vi "AFG3352XGUI.panel.vi"() -> ()   [LabVIEW 2014, in "AFG3352XGUI.lvlib"]
doc: "GUI for the AFGBase class (and its children)\n\nauthor: Dietrich Beck, GSI\nlicense: GPL"
uses:
  AFG3352XGUI.lvlib
  CSlibraries-extern/DimLVEvent/DimIndicators/DimIndicators.numericType.ctl
  CSlibraries-extern/DimLVEvent/DimIndicators/DimIndicators.anyType.ctl
  CSlibraries/UtilityLib/UtilityLib.valueStatus.ctl
  CSlibraries/UtilityLib/UtilityLib.helpType.ctl
  CSCore/CSSystem/CoreLib/CoreLib.int 2 byte array.vi
  CSCore/CSSystem/CoreLib/CoreLib.short 2 byte array.vi
  CSCore/CSSystem/CoreLib/CoreLib.short array 2 byte array.vi
  CSCore/CSSystem/CoreLib/CoreLib.double 2 byte array.vi
  CSCore/CSSystem/CoreLib/CoreLib.lvlib
  CSCore/CSObj/CSObj.lvlib
  CSlibraries/UtilityLib/UtilityLib.lvlib
  CSCore/CSApplicationBaseClasses/DeviceBase/DeviceBase.lvlib
  CSlibraries-extern/DimLVEvent/DimIndicators/DimIndicators.lvlib
  CSCore/GUIs/GOGUserGUIs/DeviceBaseGUI/DeviceBaseGUI.lvlib
panel:
  in  "actBurstMode 2":T1 caption="dic_service_numeric"
  in  "actBurstMode":T1 caption="dic_service_numeric"
  in  "actMode2":T1 caption="dic_service_numeric"
  in  "actMode":T1 caption="dic_service_numeric"
  in  "actOffset2":T1 caption="dic_service_numeric"
  in  "actAmplitude2":T1 caption="dic_service_numeric"
  in  "actPhase2":T1 caption="dic_service_numeric"
  in  "actFrequency2":T1 caption="dic_service_numeric"
  in  "Set":bool
  in  "inc":dbl
  in  "setValue":dbl
  out "Busy":bool
  out "ErrorString":string
  in  "nomValue":T1 caption="dic_service_numeric"
  in  "actOffset":T1 caption="dic_service_numeric"
  in  "actAmplitude":T1 caption="dic_service_numeric"
  in  "actPhase":T1 caption="dic_service_numeric"
  in  "actFrequency":T1 caption="dic_service_numeric"
  out "deviceIDString":string
  in  "tab":enum32{"standard", "advanced"}(tab)
  out "channelIndex":u16
  in  "nextChannel":bool
  in  "previousChannel":bool
  in  "listbox":i32(listbox)
  in  "function":u16(ring) items=["choose function", "SetFrequency", "SetAmplitude", "SetPhase", "SetDCOffset", "SetOutputEnabled", "SetMode", "SetTrigger", "SetBurstMode", "Reset"]
  in  "advancedGUI":bool
  in  "minus":bool
  in  "plus":bool
  out "loop counter":i32
  out "error out":errorcluster
  in  "error in (no error)":errorcluster
  in  "object ref":refnum<vi>
  in  "state":T1 caption="dic_service_numeric"
  in  "deviceID":T2 caption="dic_service_anyType"
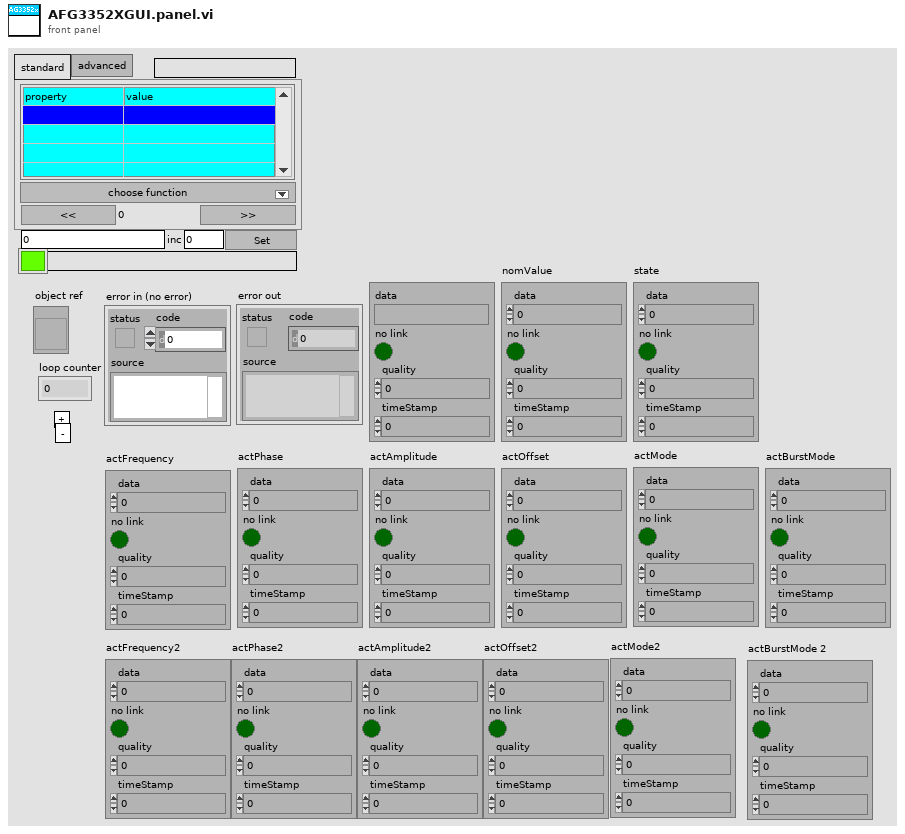
[diagram p1: front panel]
types:
  T1 = typedef "DimIndicators.lvlib/DimIndicators.numericType.ctl" = cluster{"data":dbl, "no link":bool, "quality":i32, "timeStamp":dbl}
  T2 = typedef "DimIndicators.lvlib/DimIndicators.anyType.ctl" = cluster{"data":string, "no link":bool, "quality":i32, "timeStamp":dbl}
  T3 = typedef "UtilityLib.lvlib/UtilityLib.valueStatus.ctl" = enum16{"no info available", "stand by/off", "on", "warning", "alarm/malfunction", "not implemented", "user action required", "important information", "system default", "control default", "indicator default", "button default"}
  T4 = typedef "UtilityLib.lvlib/UtilityLib.helpType.ctl" = enum16{"unknown", "menu", "description", "about", "special0", "special1", "special2"}
  T5 = typedef "CoreDefs.rawDataType.ctl" = i8[]
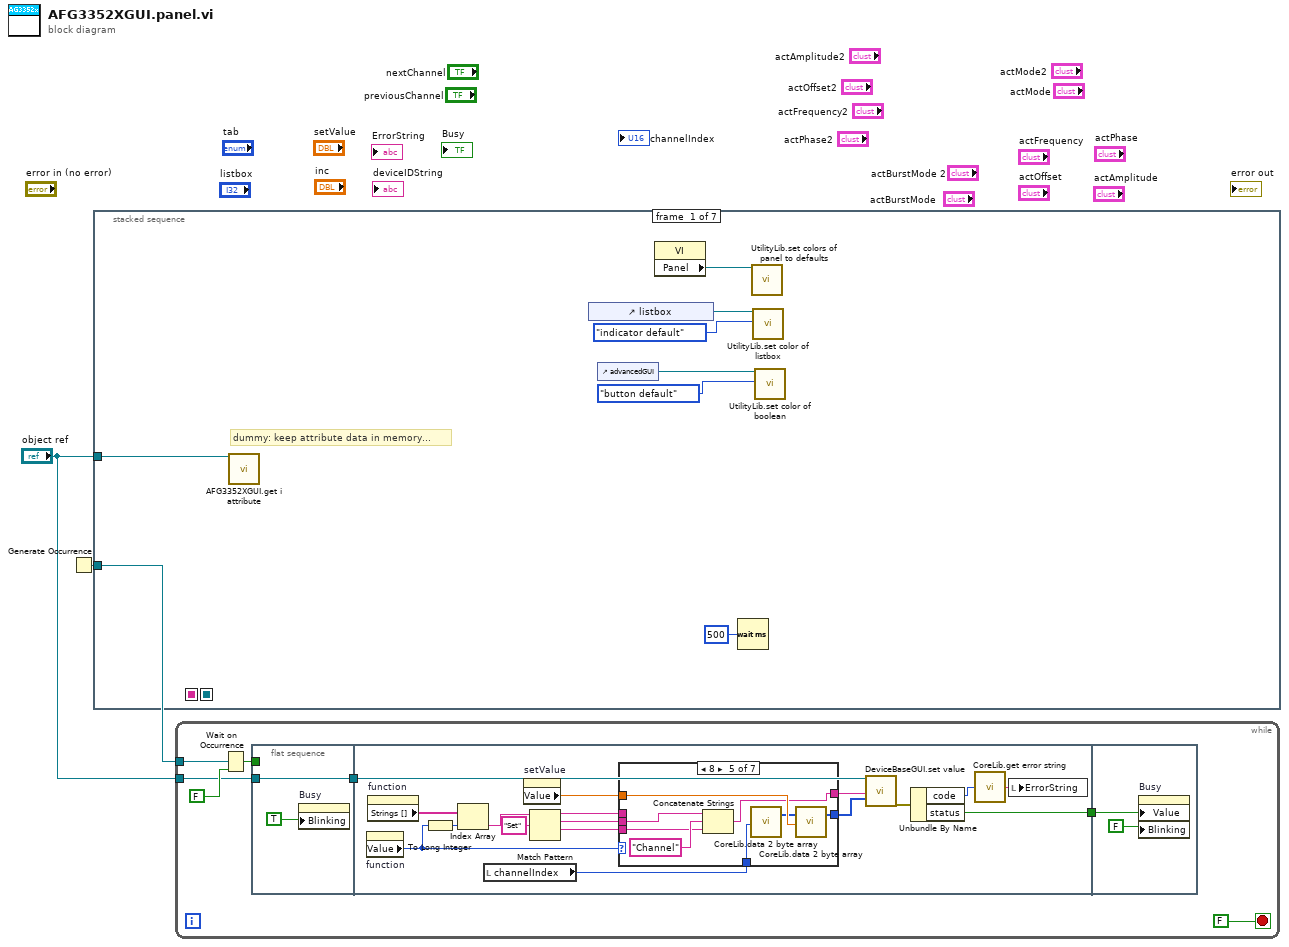
[diagram p0: block diagram]
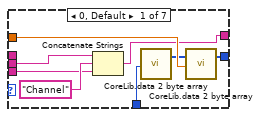
[diagram p2: hidden frame]
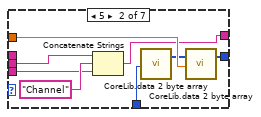
[diagram p3: hidden frame]
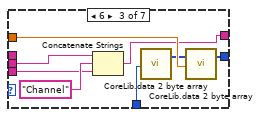
[diagram p4: hidden frame]
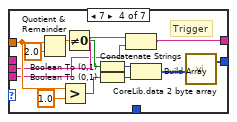
[diagram p5: hidden frame]
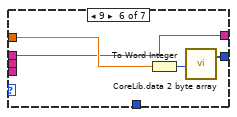
[diagram p6: hidden frame]
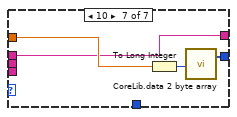
[diagram p7: hidden frame]
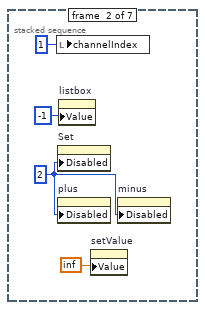
[diagram p8: hidden frame]
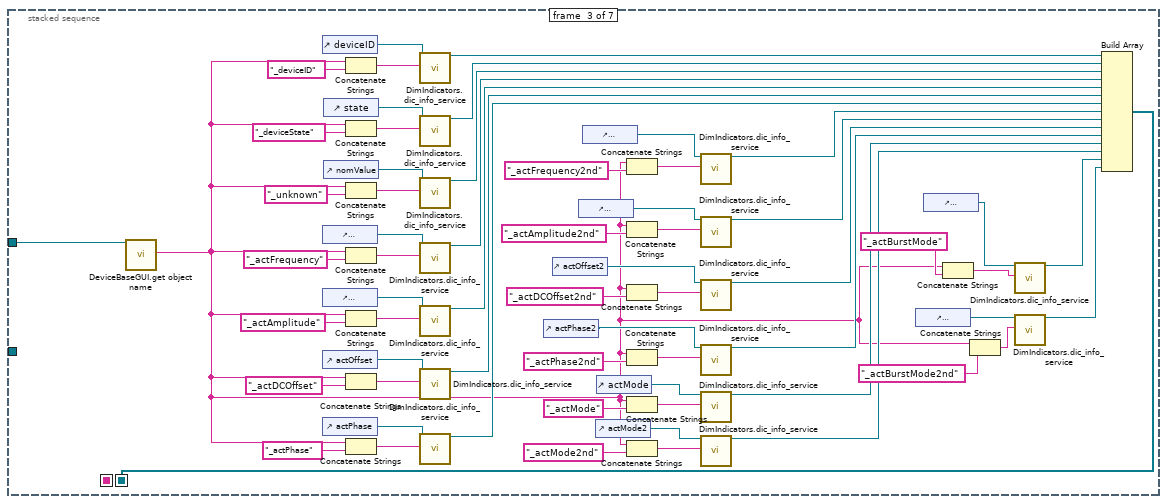
[diagram p9: hidden frame]
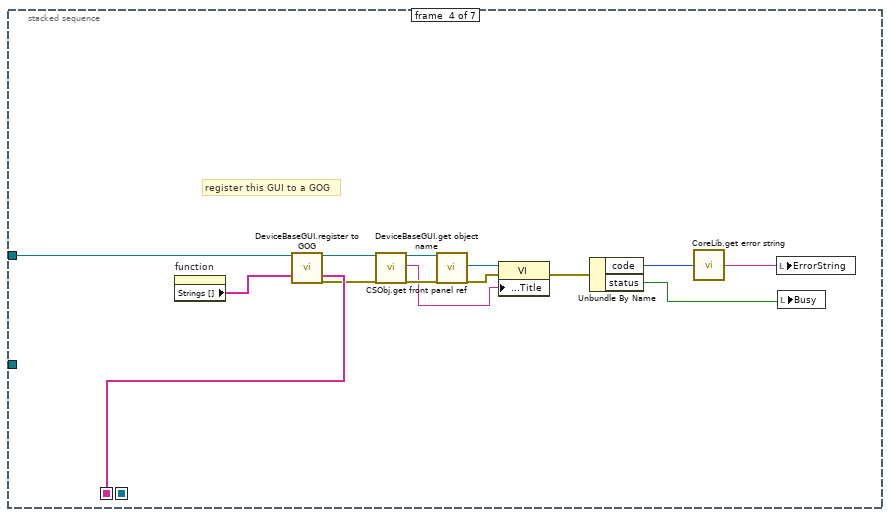
[diagram p10: hidden frame]
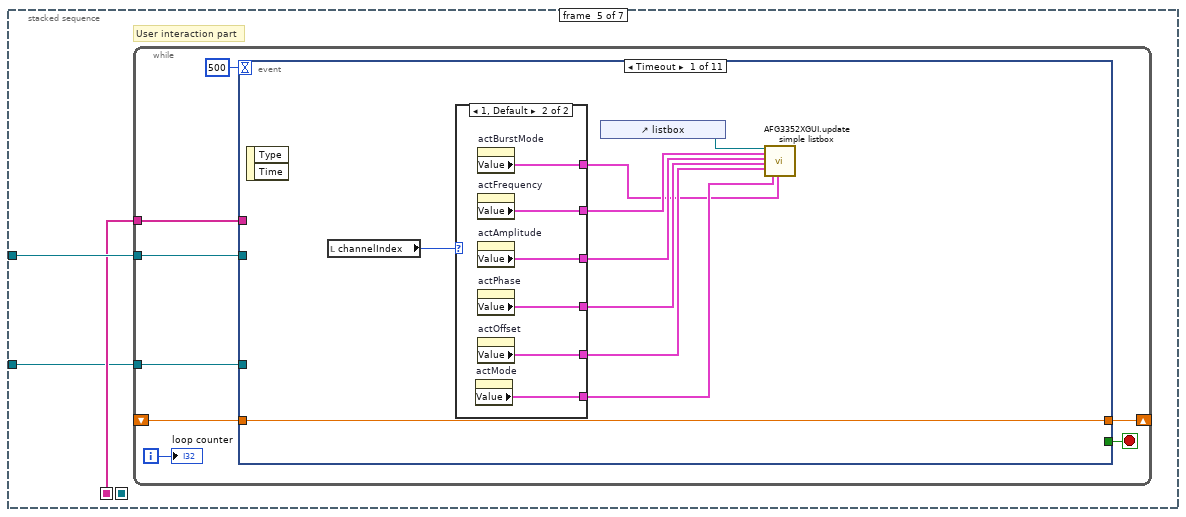
[diagram p11: hidden frame]
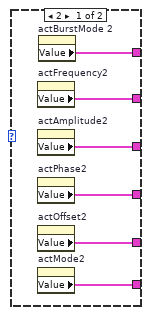
[diagram p12: hidden frame]
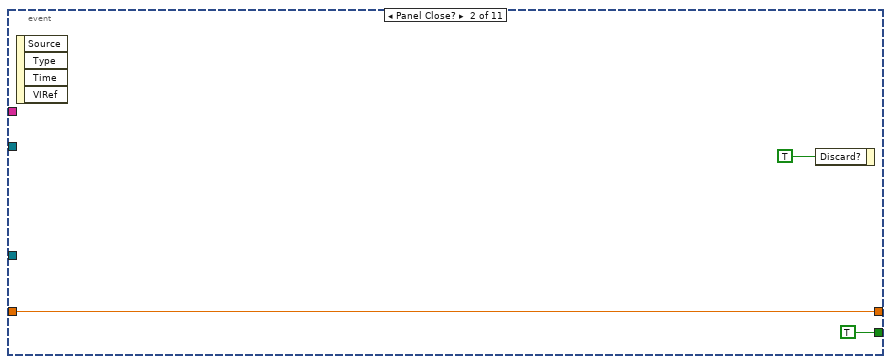
[diagram p13: hidden frame]
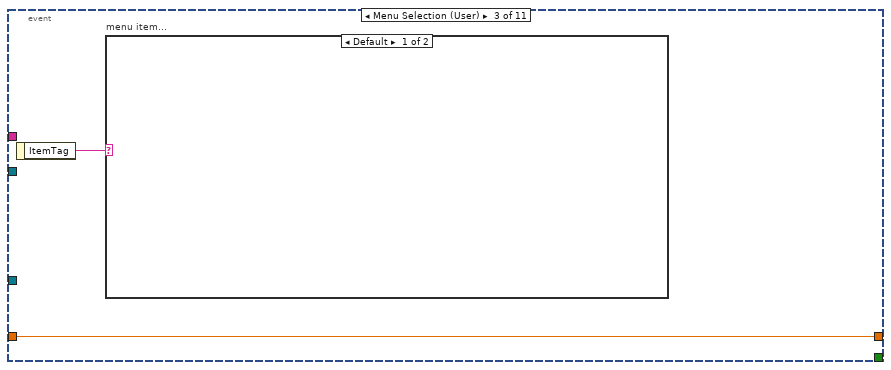
[diagram p14: hidden frame]
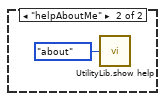
[diagram p15: hidden frame]
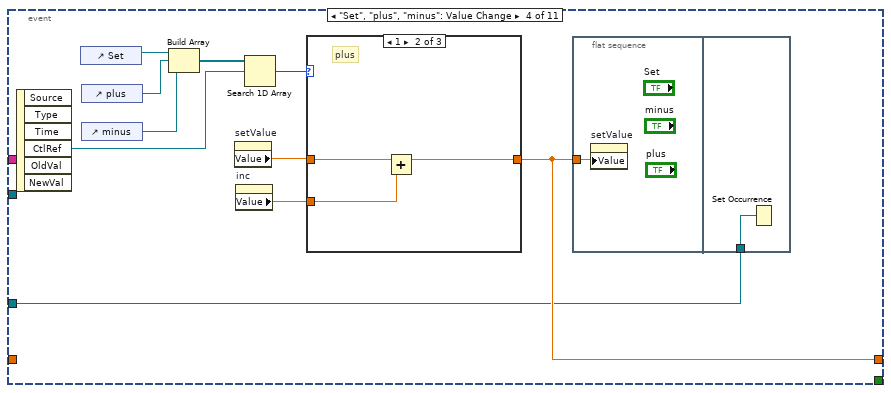
[diagram p16: hidden frame]
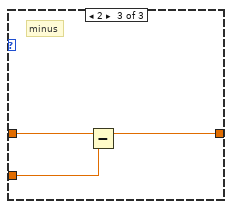
[diagram p18: hidden frame]
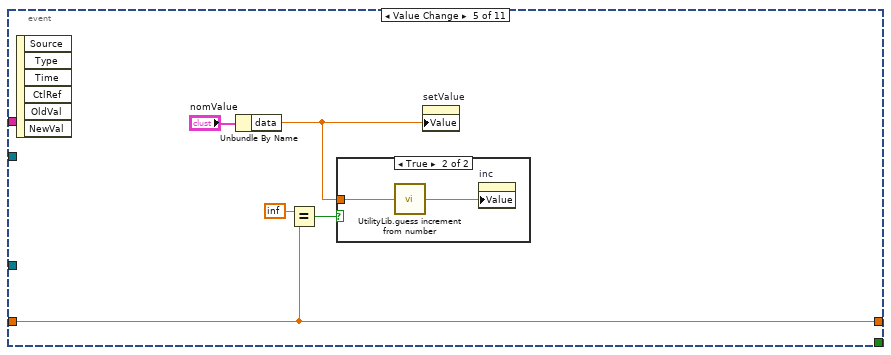
[diagram p19: hidden frame]
diagram:
  n1 = Generate Occurrence() -> (w1:refnum<k4>)
  n2 = stacked-sequence {
    seq-local: [_ _ _ w88 _ _ _] -> [_ _ _ _ w92 _ _]
    seq-local: [_ _ w47 _ _ _ _] -> [_ _ _ _ _ w216 _]
    tunnel: "object ref" -> [w3 _ w76 w78 w93 _ w218]
    tunnel: w1 -> [_ _ _ _ w91 _ _]
    frame #0 {
      # "dummy: keep attribute data in memory..."
      n3 = call "AFG3352XGUI.get i attribute.vi"("i ref in"=w3) -> ()  [unwired: 16 in, 3 out]
      n4 = control-ref of="listbox"() -> (w7:refnum<vi>)
      n5 = control-ref of="advancedGUI"() -> (w5:refnum<vi>)
      n6 = property class="VI"() -> ("Panel"=w8:refnum<vi>)  [unwired: 2 in, 2 out]
      n7 = Wait (ms)(milliseconds to wait=u32 500) -> ()  [unwired: 1 out]
      n8 = call "UtilityLib.set colors of panel to defaults.vi"("Front Panel"=w8) -> ()  [unwired: 18 in, 1 out]
      n9 = call "UtilityLib.set color of listbox.vi"("listboxRef"=w7, "valueStatus"=UtilityLib.valueStatus."indicator default") -> ()  [unwired: 17 in, 1 out]
      n10 = call "UtilityLib.set color of boolean.vi"("button"=w5, "valueStatus"=UtilityLib.valueStatus."button default") -> ()  [unwired: 17 in, 1 out]
    }
    frame #1 {
      w13 = u8 2 ("Disabled")
      n11 = local write "channelIndex"(u16 1 ("channelIndex")) -> ()
      n12 = property on="Set" class="Bool"("Disabled"=w13) -> ()  [unwired: 2 in, 2 out]
      n13 = property on="plus" class="Bool"("Disabled"=w13) -> ()  [unwired: 2 in, 2 out]
      n14 = property on="listbox" class="MCListbox (strict)"("Value"=-1 ("listbox")) -> ()  [unwired: 2 in, 2 out]
      n15 = property on="setValue" class="DigNum (strict)"("Value"=inf) -> ()  [unwired: 2 in, 2 out]
      n16 = property on="minus" class="Bool"("Disabled"=w13) -> ()  [unwired: 2 in, 2 out]
    }
    frame #2 {
      n17 = call "DeviceBaseGUI.get object name.vi"("i ref in"=w76) -> ("objectName"=w14:string)  [unwired: 16 in, 2 out]
      n18 = control-ref of="deviceID"() -> (w67:refnum<vi>)
      n19 = control-ref of="actFrequency"() -> (w58:refnum<vi>)
      n20 = control-ref of="actAmplitude"() -> (w57:refnum<vi>)
      n21 = control-ref of="actOffset"() -> (w56:refnum<vi>)
      n22 = control-ref of="actPhase"() -> (w55:refnum<vi>)
      n23 = control-ref of="state"() -> (w60:refnum<vi>)
      n24 = control-ref of="nomValue"() -> (w59:refnum<vi>)
      n25 = Concatenate Strings(w14, "_deviceID" ("string")) -> (w68:string)
      n26 = Concatenate Strings(w14, "_deviceState" ("string")) -> (w61:string)
      n27 = Concatenate Strings(w14, "_unknown" ("string")) -> (w62:string)
      n28 = Concatenate Strings(w14, "_actFrequency" ("string")) -> (w63:string)
      n29 = Concatenate Strings(w14, "_actAmplitude" ("string")) -> (w64:string)
      n30 = Concatenate Strings(w14, "_actDCOffset" ("string")) -> (w65:string)
      n31 = Concatenate Strings(w14, "_actPhase" ("string")) -> (w66:string)
      n32 = call "DimIndicators.dic_info_service.vi"("controlRef"=w67, "serviceName"=w68) -> ("controlRef out"=w54:refnum<vi>)  [unwired: 16 in, 1 out]
      n33 = call "DimIndicators.dic_info_service.vi"("controlRef"=w60, "serviceName"=w61) -> ("controlRef out"=w53:refnum<vi>)  [unwired: 16 in, 1 out]
      n34 = call "DimIndicators.dic_info_service.vi"("controlRef"=w59, "serviceName"=w62) -> ("controlRef out"=w52:refnum<vi>)  [unwired: 16 in, 1 out]
      n35 = call "DimIndicators.dic_info_service.vi"("controlRef"=w58, "serviceName"=w63) -> ("controlRef out"=w51:refnum<vi>)  [unwired: 16 in, 1 out]
      n36 = call "DimIndicators.dic_info_service.vi"("controlRef"=w57, "serviceName"=w64) -> ("controlRef out"=w50:refnum<vi>)  [unwired: 16 in, 1 out]
      n37 = call "DimIndicators.dic_info_service.vi"("controlRef"=w56, "serviceName"=w65) -> ("controlRef out"=w49:refnum<vi>)  [unwired: 16 in, 1 out]
      n38 = call "DimIndicators.dic_info_service.vi"("controlRef"=w55, "serviceName"=w66) -> ("controlRef out"=w48:refnum<vi>)  [unwired: 16 in, 1 out]
      n39 = control-ref of="actPhase2"() -> (w24:refnum<vi>)
      n40 = control-ref of="actOffset2"() -> (w23:refnum<vi>)
      n41 = control-ref of="actAmplitude2"() -> (w33:refnum<vi>)
      n42 = control-ref of="actFrequency2"() -> (w34:refnum<vi>)
      n43 = control-ref of="actMode2"() -> (w25:refnum<vi>)
      n44 = control-ref of="actMode"() -> (w26:refnum<vi>)
      n45 = Concatenate Strings(w14, "_actFrequency2nd" ("string")) -> (w42:string)
      n46 = Concatenate Strings(w14, "_actAmplitude2nd" ("string")) -> (w41:string)
      n47 = Concatenate Strings(w14, "_actDCOffset2nd" ("string")) -> (w40:string)
      n48 = Concatenate Strings(w14, "_actPhase2nd" ("string")) -> (w39:string)
      n49 = Concatenate Strings(w14, "_actMode" ("string")) -> (w31:string)
      n50 = Concatenate Strings(w14, "_actMode2nd" ("string")) -> (w29:string)
      n51 = call "DimIndicators.dic_info_service.vi"("controlRef"=w34, "serviceName"=w42) -> ("controlRef out"=w35:refnum<vi>)  [unwired: 16 in, 1 out]
      n52 = call "DimIndicators.dic_info_service.vi"("controlRef"=w33, "serviceName"=w41) -> ("controlRef out"=w36:refnum<vi>)  [unwired: 16 in, 1 out]
      n53 = call "DimIndicators.dic_info_service.vi"("controlRef"=w23, "serviceName"=w40) -> ("controlRef out"=w37:refnum<vi>)  [unwired: 16 in, 1 out]
      n54 = call "DimIndicators.dic_info_service.vi"("controlRef"=w24, "serviceName"=w39) -> ("controlRef out"=w38:refnum<vi>)  [unwired: 16 in, 1 out]
      n55 = call "DimIndicators.dic_info_service.vi"("controlRef"=w26, "serviceName"=w31) -> ("controlRef out"=w28:refnum<vi>)  [unwired: 16 in, 1 out]
      n56 = call "DimIndicators.dic_info_service.vi"("controlRef"=w25, "serviceName"=w29) -> ("controlRef out"=w27:refnum<vi>)  [unwired: 16 in, 1 out]
      n57 = control-ref of="actBurstMode 2"() -> (w19:refnum<vi>)
      n58 = control-ref of="actBurstMode"() -> (w20:refnum<vi>)
      n59 = Concatenate Strings(w14, "_actBurstMode" ("string")) -> (w16:string)
      n60 = Concatenate Strings(w14, "_actBurstMode2nd" ("string")) -> (w18:string)
      n61 = call "DimIndicators.dic_info_service.vi"("controlRef"=w20, "serviceName"=w16) -> ("controlRef out"=w22:refnum<vi>)  [unwired: 16 in, 1 out]
      n62 = call "DimIndicators.dic_info_service.vi"("controlRef"=w19, "serviceName"=w18) -> ("controlRef out"=w21:refnum<vi>)  [unwired: 16 in, 1 out]
      n63 = Build Array(w54, w53, w52, w51, w50, w49, w48, w35, w36, w37, w38, w28, w27, w22, w21) -> (w47:refnum<vi>[])
    }
    frame #3 {
      # "register this GUI to a GOG"
      n64 = property on="function" class="Ring (strict)"() -> ("Strings []"=w89:string[])  [unwired: 2 in, 2 out]
      n65 = call "DeviceBaseGUI.register to GOG.vi"("i ref in"=w78, "myMethods"=w89) -> ("i ref out"=w86:refnum<vi>, "configuredMethods"=w88:string[], "error out"=w87:errorcluster)  [unwired: 15 in]
      n66 = call "DeviceBaseGUI.get object name.vi"("i ref in"=w86, "error in (no error)"=w87) -> ("i ref out"=w85:refnum<vi>, "objectName"=w77:string, "error out"=w84:errorcluster)  [unwired: 15 in]
      n67 = call "CSObj.get front panel ref.vi"("i ref in"=w85, "error in (no error)"=w84) -> ("frontPanelRef"=w90:refnum<vi>, "error out"=w80:errorcluster)  [unwired: 15 in, 1 out]
      n68 = property class="VI"(reference=w90, error in=w80, "Front Panel Window:Title"=w77) -> (error out=w79:errorcluster)  [unwired: 1 out]
      n69 = Unbundle By Name(w79) -> ("code"=w83:i32, "status"=w81:bool)
      n70 = call "CoreLib.get error string.vi"("Error Code"=w83) -> ("Error String"=w82:string)
      n71 = local write "ErrorString"(w82) -> ()
      n72 = local write "Busy"(w81) -> ()
    }
    frame #4 {
      # "User interaction part"
      n73 = while {
        tunnel: w93 -> [w100]
        shift-right: [w97] -> _
        shift-left: _ -> [w98]
        tunnel: w92 -> [w96]
        tunnel: w91 -> [w95]
        i -> [w101]
        stop <- w94 stop-if-true
        n74 = event shown="[0] Timeout" {
          selector: _ -> [_ _ _ _ _ _ _ _ _ _ _]
          dyn-events: _ -> [_ _ _ _ _ _ _ _ _ _ _]
          timeout: 500 -> [_ _ _ _ _ _ _ _ _ _ _]
          tunnel: w100 -> [_ _ _ _ _ w165 _ _ w195 _ _]
          tunnel: [w110 w125 w127 w130 w150 w156 w185 w191 w194 w205 w214] -> w97
          tunnel: w98 -> [w110 w125 w127 _ w150 _ w185 w191 w194 w205 w214]
          tunnel: w96 -> [_ _ _ _ _ w163 _ _ _ _ _]
          tunnel: w95 -> [_ _ _ w129 _ _ _ _ _ _ _]
          tunnel: [_ TRUE ("Discard?") _ _ _ _ _ _ _ _ _] -> w94
          event Timeout {
            n75 = event-data() -> ()  [unwired: 1 in, 2 out]
            n76 = local read "channelIndex"() -> (w104:u16)
            n77 = case shown="1, Default" w104 {
              tunnel: [w116 w122] -> w108
              tunnel: [w115 w121] -> w107
              tunnel: [w114 w120] -> w106
              tunnel: [w113 w119] -> w105
              tunnel: [w112 w118] -> w103
              tunnel: [w111 w117] -> w102
              frame 2 {
                n78 = property on="actFrequency2" class="Clust (strict)"() -> ("Value"=w116:T1)  [unwired: 2 in, 2 out]
                n79 = property on="actAmplitude2" class="Clust (strict)"() -> ("Value"=w115:T1)  [unwired: 2 in, 2 out]
                n80 = property on="actPhase2" class="Clust (strict)"() -> ("Value"=w114:T1)  [unwired: 2 in, 2 out]
                n81 = property on="actOffset2" class="Clust (strict)"() -> ("Value"=w113:T1)  [unwired: 2 in, 2 out]
                n82 = property on="actMode2" class="Clust (strict)"() -> ("Value"=w112:T1)  [unwired: 2 in, 2 out]
                n83 = property on="actBurstMode 2" class="Clust (strict)"() -> ("Value"=w111:T1)  [unwired: 2 in, 2 out]
              }
              frame 1, Default {
                n84 = property on="actMode" class="Clust (strict)"() -> ("Value"=w118:T1)  [unwired: 2 in, 2 out]
                n85 = property on="actBurstMode" class="Clust (strict)"() -> ("Value"=w117:T1)  [unwired: 2 in, 2 out]
                n86 = property on="actFrequency" class="Clust (strict)"() -> ("Value"=w122:T1)  [unwired: 2 in, 2 out]
                n87 = property on="actAmplitude" class="Clust (strict)"() -> ("Value"=w121:T1)  [unwired: 2 in, 2 out]
                n88 = property on="actPhase" class="Clust (strict)"() -> ("Value"=w120:T1)  [unwired: 2 in, 2 out]
                n89 = property on="actOffset" class="Clust (strict)"() -> ("Value"=w119:T1)  [unwired: 2 in, 2 out]
              }
            }
            n90 = control-ref of="listbox"() -> (w109:refnum<vi>)
            n91 = call "AFG3352XGUI.update simple listbox.vi"("listbox"=w109, "actFrequency"=w108, "actAmplitude"=w107, "actPhase"=w106, "actOffset"=w105, "actMode"=w103, "actBurstMode"=w102) -> ()  [unwired: 12 in, 1 out]
          }
          event Panel Close? {
            n92 = event-data() -> ()  [unwired: 1 in, 4 out]
            n93 = event-data("Discard?"=TRUE) -> ()  [unwired: 1 in, 1 out]
          }
          event Menu Selection (User) {
            n94 = event-data() -> ("ItemTag"=w126:string)  [unwired: 1 in]
            n95 = case "menu item..." shown="Default" w126 {
              frame Default {
              }
              frame "helpAboutMe" {
                n96 = call "UtilityLib.show help.vi"("helpType"=UtilityLib.helpType."about") -> ()
              }
            }
          }
          event "Set", "plus", "minus": Value Change {
            n97 = event-data() -> ("CtlRef"=w134:refnum<vi>)  [unwired: 1 in, 5 out]
            n98 = control-ref of="Set"() -> (w138:refnum<vi>)
            n99 = control-ref of="plus"() -> (w137:refnum<vi>)
            n100 = control-ref of="minus"() -> (w136:refnum<vi>)
            n101 = Build Array(w138, w137, w136) -> (w135:refnum<vi>[])
            n102 = property on="setValue" class="DigNum (strict)"() -> ("Value"=w131:dbl)  [unwired: 2 in, 2 out]
            n103 = property on="inc" class="DigNum (strict)"() -> ("Value"=w132:dbl)  [unwired: 2 in, 2 out]
            n104 = Search 1D Array(1D array=w135, element=w134) -> (index of element=w133:i32)  [unwired: 1 in]
            n105 = case shown="1" w133 {
              tunnel: [w141 w143 w146] -> w130
              tunnel: w131 -> [w141 w144 w147]
              tunnel: w132 -> [_ w142 w145]
              frame 0, Default {
                # "set"
              }
              frame 1 {
                # "plus"
                n106 = Add(x=w144, y=w142) -> (x+y=w143:dbl)
              }
              frame 2 {
                # "minus"
                n107 = Subtract(x=w147, y=w145) -> (x-y=w146:dbl)
              }
            }
            n108 = flat-sequence {
              tunnel: w130 -> [w139]
              tunnel: w129 -> [w140]
              frame #0 {
                n109 = property on="setValue" class="DigNum (strict)"("Value"=w139) -> ()  [unwired: 2 in, 2 out]
              }
              frame #1 {
                n110 = Set Occurrence(w140) -> ()
              }
            }
          }
          event Value Change {
            n111 = event-data() -> ()  [unwired: 1 in, 6 out]
            n112 = Unbundle By Name("nomValue") -> ("data"=w152:dbl)
            n113 = Equal?(x=inf, y=w150) -> (x = y?=w148:bool)
            n114 = case shown="True" w148 {
              tunnel: w152 -> [_ w154]
              frame False {
              }
              frame True {
                n115 = call "UtilityLib.guess increment from number.vi"("number"=w154) -> ("increment"=w153:dbl)
                n116 = property on="inc" class="DigNum (strict)"("Value"=w153) -> ()  [unwired: 2 in, 2 out]
              }
            }
            n117 = property on="setValue" class="DigNum (strict)"("Value"=w152) -> ()  [unwired: 2 in, 2 out]
          }
          event "function": Value Change {
            w156 = inf
            n118 = event-data() -> ()  [unwired: 1 in, 6 out]
            n119 = property on="function" class="Ring (strict)"() -> ("Strings []"=w164:string[])  [unwired: 2 in, 2 out]
            n120 = property on="setValue" class="DigNum (strict)"("Value"=w156) -> (error out=w160:errorcluster)  [unwired: 2 in, 1 out]
            n121 = control-ref of="nomValue"() -> (w157:refnum<vi>)
            n122 = To Long Integer(number="function") -> (32bit integer=w155:i32)
            n123 = Index Array(array=w164, index=w155) -> (element=w162:string)
            n124 = call "DimIndicators.dic_release_service.vi"("controlRef"=w157) -> ("error out"=w158:errorcluster)  [unwired: 18 in]
            n125 = Search 1D Array(1D array=w163, element=w162) -> (index of element=w161:i32)  [unwired: 1 in]
            n126 = case "method configured?" shown="0, Default" w161 {
              tunnel: w165 -> [w172 _]
              tunnel: "function" -> [w171 _]
              tunnel: w158 -> [w169 _]
              tunnel: w160 -> [_ _]
              tunnel: w157 -> [w168 _]
              frame 0, Default {
                w170 = u8 0 ("Disabled")
                n127 = case shown="6" w171 {
                  tunnel: ["_nomFrequency" "_nomAmplitude" "_nomPhase" "_nomDCOffset" "_nomOutputEnabled" "_nomWaveformType" "unknown"] -> w173
                  frame 1 {
                  }
                  frame 2 {
                  }
                  frame 3 {
                  }
                  frame 4 {
                  }
                  frame 6 {
                  }
                  frame 7 {
                  }
                  frame 0, Default {
                  }
                }
                n128 = call "DeviceBaseGUI.get object name.vi"("i ref in"=w172) -> ("objectName"=w166:string)  [unwired: 16 in, 2 out]
                n129 = Concatenate Strings(w166, w173) -> (w167:string)
                n130 = property on="Set" class="Bool"("Disabled"=w170) -> ()  [unwired: 2 in, 2 out]
                n131 = property on="plus" class="Bool"("Disabled"=w170) -> ()  [unwired: 2 in, 2 out]
                n132 = call "DimIndicators.dic_info_service.vi"("controlRef"=w168, "serviceName"=w167, "error in (no error)"=w169) -> ()  [unwired: 15 in, 2 out]
                n133 = property on="minus" class="Bool"("Disabled"=w170) -> ()  [unwired: 2 in, 2 out]
              }
              frame -1 {
                w181 = u8 2 ("Disabled")
                n134 = property on="Set" class="Bool"("Disabled"=w181) -> ()  [unwired: 2 in, 2 out]
                n135 = property on="plus" class="Bool"("Disabled"=w181) -> ()  [unwired: 2 in, 2 out]
                n136 = property on="minus" class="Bool"("Disabled"=w181) -> ()  [unwired: 2 in, 2 out]
              }
            }
          }
          event Value Change {
            n137 = event-data() -> ()  [unwired: 1 in, 6 out]
            n138 = Unbundle By Name("deviceID") -> ("data"=w184:string)
            n139 = call "UtilityLib.remove white spaces.vi"("string with blanks"=w184) -> ("string without white spaces"=w183:string)  [unwired: 14 in, 4 out]
            n140 = property on="deviceIDString" class="Str"("Value"=w183) -> ()  [unwired: 2 in, 2 out]
          }
          event Value Change {
            n141 = event-data() -> ()  [unwired: 1 in, 6 out]
            n142 = Unbundle By Name("state") -> ("no link"=w192:bool, "data"=w188:dbl)
            n143 = call "DeviceBase.device state 2 value status.vi"("deviceState"=w188, "no link"=w192) -> ("valueStatus"=w190:T3)
            n144 = call "UtilityLib.Sixcolor.vi"("State"=w190) -> ("elementBackground"=w189:u32, "elementText"=w186:u32)  [unwired: 2 in, 2 out]
            n145 = property on="deviceIDString" class="Str"("Text.BGColor"=w189, "Text.TextColor"=w186) -> ()  [unwired: 2 in, 2 out]
          }
          event "advancedGUI": Value Change {
            n146 = event-data() -> ()  [unwired: 1 in, 6 out]
            n147 = call "DeviceBaseGUI.get object name.vi"("i ref in"=w195) -> ("objectName"=w193:string)  [unwired: 16 in, 2 out]
            n148 = call "DeviceBase.create advanced GUI.vi"("Object"=w193) -> ()  [unwired: 17 in, 2 out]
          }
          event "nextChannel": Value Change {
            n149 = event-data() -> ()  [unwired: 1 in, 6 out]
            n150 = control-ref of="listbox"() -> (w203:refnum<vi>)
            n151 = property on="actMode2" class="Clust (strict)"() -> ("Value"=w197:T1)  [unwired: 2 in, 2 out]
            n152 = property on="actFrequency2" class="Clust (strict)"() -> ("Value"=w202:T1)  [unwired: 2 in, 2 out]
            n153 = property on="actAmplitude2" class="Clust (strict)"() -> ("Value"=w201:T1)  [unwired: 2 in, 2 out]
            n154 = property on="actPhase2" class="Clust (strict)"() -> ("Value"=w200:T1)  [unwired: 2 in, 2 out]
            n155 = property on="actOffset2" class="Clust (strict)"() -> ("Value"=w199:T1)  [unwired: 2 in, 2 out]
            n156 = property on="actBurstMode 2" class="Clust (strict)"() -> ("Value"=w196:T1)  [unwired: 2 in, 2 out]
            n157 = call "AFG3352XGUI.update simple listbox.vi"("listbox"=w203, "actFrequency"=w202, "actAmplitude"=w201, "actPhase"=w200, "actOffset"=w199, "actMode"=w197, "actBurstMode"=w196) -> ()  [unwired: 12 in, 1 out]
            n158 = local write "channelIndex"(u16 2 ("channelIndex")) -> ()
            n159 = local write "nextChannel"(FALSE ("nextChannel")) -> ()
          }
          event "previousChannel": Value Change {
            n160 = event-data() -> ()  [unwired: 1 in, 6 out]
            n161 = control-ref of="listbox"() -> (w213:refnum<vi>)
            n162 = property on="actMode" class="Clust (strict)"() -> ("Value"=w207:T1)  [unwired: 2 in, 2 out]
            n163 = property on="actFrequency" class="Clust (strict)"() -> ("Value"=w212:T1)  [unwired: 2 in, 2 out]
            n164 = property on="actAmplitude" class="Clust (strict)"() -> ("Value"=w211:T1)  [unwired: 2 in, 2 out]
            n165 = property on="actPhase" class="Clust (strict)"() -> ("Value"=w210:T1)  [unwired: 2 in, 2 out]
            n166 = property on="actOffset" class="Clust (strict)"() -> ("Value"=w209:T1)  [unwired: 2 in, 2 out]
            n167 = property on="actBurstMode" class="Clust (strict)"() -> ("Value"=w206:T1)  [unwired: 2 in, 2 out]
            n168 = call "AFG3352XGUI.update simple listbox.vi"("listbox"=w213, "actFrequency"=w212, "actAmplitude"=w211, "actPhase"=w210, "actOffset"=w209, "actMode"=w207, "actBurstMode"=w206) -> ()  [unwired: 12 in, 1 out]
            n169 = local write "previousChannel"(FALSE ("previousChannel")) -> ()
            n170 = local write "channelIndex"(u16 1 ("channelIndex")) -> ()
          }
        }
        "loop counter" <- w101
      }
    }
    frame #5 {
      n171 = for {
        tunnel: w216 -> [w217] mode=indexing
        n172 = call "DimIndicators.dic_release_service.vi"("controlRef"=w217) -> ()  [unwired: 18 in, 1 out]
      }
    }
    frame #6 {
      n173 = call "DeviceBaseGUI.close panel.vi"("i ref in"=w218) -> ()  [unwired: 17 in, 2 out]
    }
  }
  n174 = while {
    tunnel: w1 -> [w223]
    tunnel: "object ref" -> [w220]
    stop <- FALSE stop-if-true
    n175 = Wait on Occurrence(1:FALSE ("ignore previous (T)"), 2:w223) -> (0:w222:bool)  [unwired: 1 in]
    n176 = flat-sequence {
      tunnel: w222 -> [_]
      tunnel: [w226] -> w221
      tunnel: w220 -> [w226]
      tunnel: w221 -> [w238]
      tunnel: [w236] -> w219
      tunnel: w219 -> [w298]
      frame #0 {
        n177 = property on="Busy" class="Bool (strict)"("Blinking"=TRUE) -> ()  [unwired: 2 in, 2 out]
      }
      frame #1 {
        n178 = property on="function" class="Ring (strict)"() -> ("Value"=w244:u16)  [unwired: 2 in, 2 out]
        n179 = property on="function" class="Ring (strict)"() -> ("Strings []"=w242:string[])  [unwired: 2 in, 2 out]
        n180 = To Long Integer(number=w244) -> (32bit integer=w235:i32)
        n181 = Index Array(array=w242, index=w235) -> (element=w234:string)
        n182 = local read "channelIndex"() -> (w232:u16)
        n183 = property on="setValue" class="DigNum (strict)"() -> ("Value"=w237:dbl)  [unwired: 2 in, 2 out]
        n184 = Match Pattern(string=w234, regular expression="Set") -> (before substring=w230:string, match substring=w231:string, after substring=w229:string)  [unwired: 1 in, 1 out]
        n185 = case shown="8" w244 {
          tunnel: [w252 w260 w268 w281 w289 w293 w297] -> w243
          tunnel: w237 -> [w251 w259 w267 w273 w288 w292 w296]
          tunnel: w232 -> [w249 w257 w265 _ w286 _ _]
          tunnel: w231 -> [w247 w255 w263 w270 w284 _ _]
          tunnel: w230 -> [_ _ _ _ _ w290 w294]
          tunnel: w229 -> [w246 w254 w262 w269 w283 _ _]
          tunnel: [w245 w253 w261 w271 w282 w290 w294] -> w228
          frame 0, Default {
            n186 = Concatenate Strings(w247, "Channel" ("string"), w246) -> (w245:string)
            n187 = call-poly "CoreLib.data 2 byte array.vi"("i32"=w249) -> ("byteArray out"=w250:T5)  [unwired: 18 in]
            n188 = call-poly "CoreLib.data 2 byte array.vi"("byteArray"=w250, "f64"=w251) -> ("byteArray out"=w252:T5)  [unwired: 17 in]
          }
          frame 5 {
            n189 = Concatenate Strings(w255, "Channel" ("string"), w254) -> (w253:string)
            n190 = call-poly "CoreLib.data 2 byte array.vi"("i32"=w257) -> ("byteArray out"=w258:T5)  [unwired: 18 in]
            n191 = call-poly "CoreLib.data 2 byte array.vi"("byteArray"=w258, "i16"=w259) -> ("byteArray out"=w260:T5)  [unwired: 17 in]
          }
          frame 6 {
            n192 = Concatenate Strings(w263, "Channel" ("string"), w262) -> (w261:string)
            n193 = call-poly "CoreLib.data 2 byte array.vi"("i32"=w265) -> ("byteArray out"=w266:T5)  [unwired: 18 in]
            n194 = call-poly "CoreLib.data 2 byte array.vi"("byteArray"=w266, "i32"=w267) -> ("byteArray out"=w268:T5)  [unwired: 17 in]
          }
          frame 7 {
            # "Trigger"
            n195 = Quotient & Remainder(x=w273, y=2.0) -> (x-y*floor(x/y)=w276:dbl)  [unwired: 1 out]
            n196 = Greater?(x=w273, y=1.0) -> (0:w274:bool)
            n197 = Not Equal To 0?(x=w276) -> (x != 0?=w275:bool)
            n198 = Boolean To (0,1)(Boolean=w275) -> (0, 1=w279:i16)
            n199 = Boolean To (0,1)(Boolean=w274) -> (0, 1=w278:i16)
            n200 = Concatenate Strings(w270, w269) -> (w271:string)
            n201 = Build Array(w279, w278) -> (w280:i16[])
            n202 = call-poly "CoreLib.data 2 byte array.vi"("[i16]"=w280) -> ("byteArray out"=w281:T5)  [unwired: 18 in]
          }
          frame 8 {
            n203 = Concatenate Strings(w284, "Channel" ("string"), w283) -> (w282:string)
            n204 = call-poly "CoreLib.data 2 byte array.vi"("i32"=w286) -> ("byteArray out"=w287:T5)  [unwired: 18 in]
            n205 = call-poly "CoreLib.data 2 byte array.vi"("byteArray"=w287, "i32"=w288) -> ("byteArray out"=w289:T5)  [unwired: 17 in]
          }
          frame 9 {
            n206 = To Word Integer(number=w292) -> (16bit integer=w291:i16)
            n207 = call-poly "CoreLib.data 2 byte array.vi"("i16"=w291) -> ("byteArray out"=w293:T5)  [unwired: 18 in]
          }
          frame 10 {
            n208 = To Long Integer(number=w296) -> (32bit integer=w295:i32)
            n209 = call-poly "CoreLib.data 2 byte array.vi"("i32"=w295) -> ("byteArray out"=w297:T5)  [unwired: 18 in]
          }
        }
        n210 = call "DeviceBaseGUI.set value.vi"("i ref in"=w238, "methodName"=w228, "byteArray"=w243) -> ("error out"=w240:errorcluster)  [unwired: 15 in, 1 out]
        n211 = Unbundle By Name(w240) -> ("code"=w241:i32, "status"=w236:bool)
        n212 = call "CoreLib.get error string.vi"("Error Code"=w241) -> ("Error String"=w239:string)
        n213 = local write "ErrorString"(w239) -> ()
      }
      frame #2 {
        n214 = property on="Busy" class="Bool (strict)"("Value"=w298, "Blinking"=FALSE) -> ()  [unwired: 2 in, 2 out]
      }
    }
  }
